vi "Extras_1SDI.vi"(8 "Scope+Safety":T3={"Safety First"={"lim reset"=FALSE, "no limit"=FALSE, "pos slew rate * dt"=100, "neg slew rate * dt"=-100, "Count(Ticks)"=0}, "Scope IPs"={"Trigger Direction"=enum."minus-plus", "Trigger Delay (ms)"=0.0, "Aquisition Rate (kHz)"=4000.0, "Trigger Offset (V)"=0.0, "Scale Offset"={"Scaling"={"Error signal"=1, "Output"=1, "DC Monitor"=1, "Threshold"=1}, "Offset"={"Error Signal"=0, "Output"=0, "DC Monitor"=0, "Threshold"=0}}}}, 11 "Extras 1SDI":T4={"Error Bit Shift "={"EPR BS"=0, "HD A x"=0, "HD A p"=0, "HD B x"=0, "HD B p"=0, "HD C x"=0, "HD C p"=0}, "I Max value"=20000, "Scan Offset"={"EPR BS"=0.0, "HD A"=0.0, "HD B"=0.0, "HD C"=0.0}, "Scan Ampl.\n     (mV)"={"EPR BS"=0.0, "HD A"=0.0, "HD B"=0.0, "HD C"=0.0}, "Scan-PII thresh"={"EPR BS"=0, "Homodyne A"=0, "Homodyne B"=0, "Homodyne C"=0}, "Re-Scan thresh"={"EPR BS"=1000, "Homodyne A"=1000, "Homodyne B"=1000, "Homodyne C"=0}, "Post-Offset"={"HD A x"=0.0, "HD A p"=0.0, "HD B x"=0.0, "HD B p"=0.0, "HD C x"=0.0, "HD C p"=0.0}}) -> (0 "Extras Homodyne C":T1, 1 "Extras Homodyne B":T1, 2 "Extras Homodyne A":T1, 3 "Extras EPR BS":T2)   [LabVIEW 2013]
uses:
  Strict Type Defs/Extras 1SDI.ctl
  Strict Type Defs/Double ISDI control.ctl
  Strict Type Defs/I16 1SDI Control.ctl
  Strict Type Defs/Scope and Safety.ctl
  Strict Type Defs/Extras PII 1SDI.ctl
  Strict Type Defs/Extras PII 1SDI HD.ctl
panel:
  in  "Extras HD C":T1
  in  "Extras HD B":T1
  in  "Extras HD A":T1
  in  "Extras PII 1SDI":T2
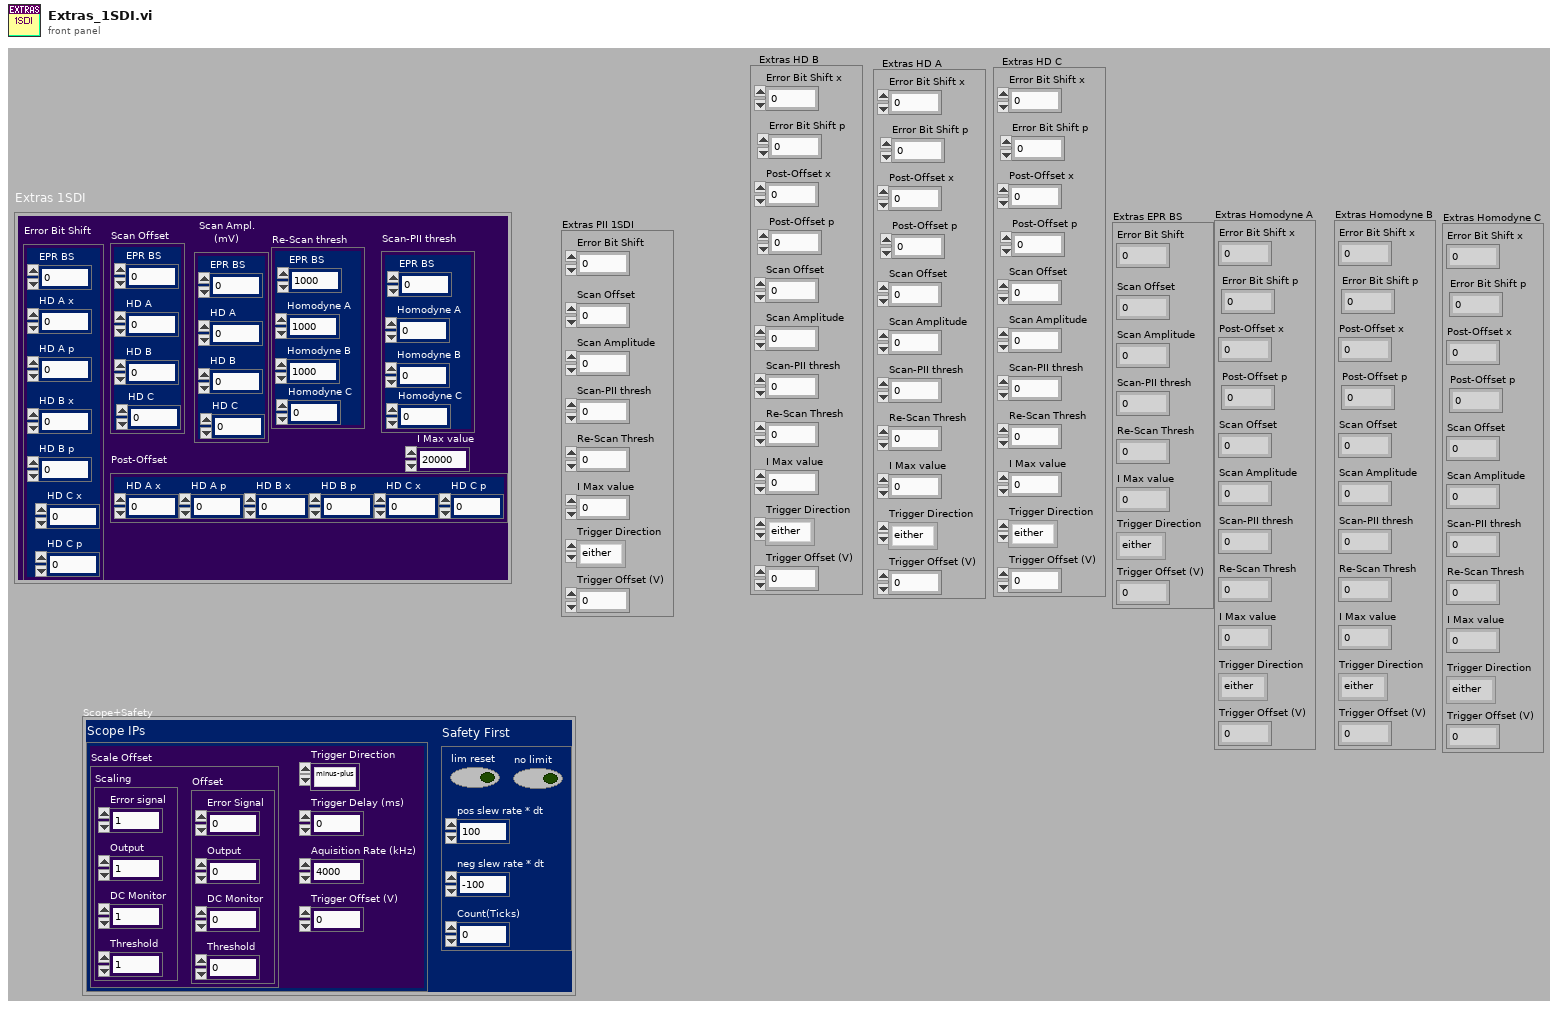
[diagram p1: front panel]
types:
  T1 = typedef "Extras PII 1SDI HD.ctl" = cluster{"Error Bit Shift p":i16, "Scan Offset":dbl, "Scan Amplitude":dbl, "Scan-PII thresh":i16, "Re-Scan Thresh":i16, "I Max value":i32, "Trigger Direction":enum8{"either", "minus-plus", "plus-minus"}, "Trigger Offset (V)":dbl, "Error Bit Shift x":i16, "Post-Offset p":dbl, "Post-Offset x":dbl}
  T2 = typedef "Extras PII 1SDI.ctl" = cluster{"Error Bit Shift":i16, "Scan Offset":dbl, "Scan Amplitude":dbl, "Scan-PII thresh":i16, "Re-Scan Thresh":i16, "I Max value":i32, "Trigger Direction":enum8{"either", "minus-plus", "plus-minus"}, "Trigger Offset (V)":dbl}
  T3 = typedef "Scope and Safety.ctl" = cluster{"Safety First":cluster{"lim reset":bool, "no limit":bool, "pos slew rate * dt":i16, "neg slew rate * dt":i16, "Count(Ticks)":u32}, "Scope IPs":cluster{"Trigger Direction":enum8{"either", "minus-plus", "plus-minus"}, "Trigger Delay (ms)":dbl, "Aquisition Rate (kHz)":dbl, "Trigger Offset (V)":dbl, "Scale Offset":cluster{"Scaling":cluster{"Error signal":i16, "Output":i16, "DC Monitor":i16, "Threshold":i16}, "Offset":cluster{"Error Signal":i16, "Output":i16, "DC Monitor":i16, "Threshold":i16}}}}
  T4 = typedef "Extras 1SDI.ctl" = cluster{"Error Bit Shift ":cluster{"EPR BS":i16, "HD A x":i16, "HD A p":i16, "HD B x":i16, "HD B p":i16, "HD C x":i16, "HD C p":i16}, "I Max value":i32, "Scan Offset":T5, "Scan Ampl.\n     (mV)":T5, "Scan-PII thresh":T6, "Re-Scan thresh":T6, "Post-Offset":cluster{"HD A x":dbl, "HD A p":dbl, "HD B x":dbl, "HD B p":dbl, "HD C x":dbl, "HD C p":dbl}}
  T5 = typedef "Double ISDI control.ctl" = cluster{"EPR BS":dbl, "HD A":dbl, "HD B":dbl, "HD C":dbl}
  T6 = typedef "I16 1SDI Control.ctl" = cluster{"EPR BS":i16, "Homodyne A":i16, "Homodyne B":i16, "Homodyne C":i16}
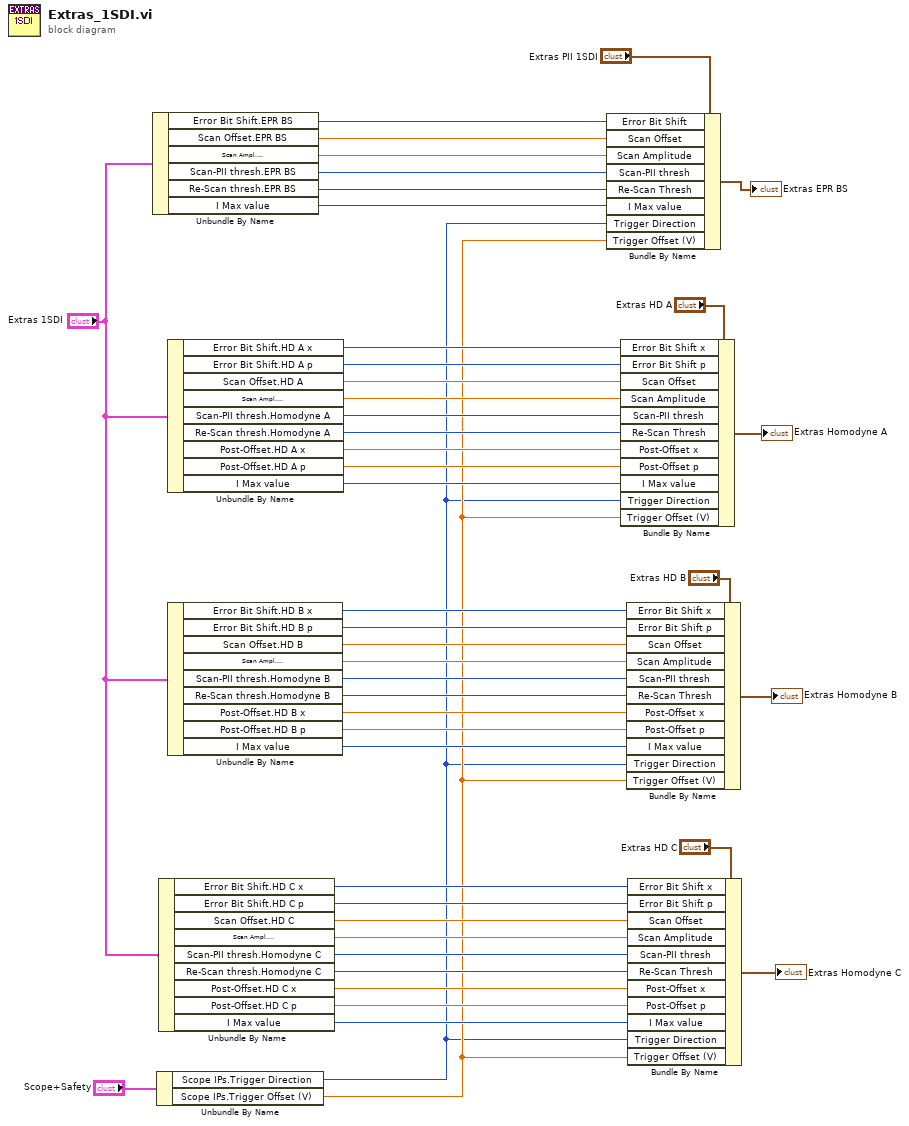
[diagram p0: block diagram]
diagram:
  n1 = Unbundle By Name("Extras 1SDI") -> ("Error Bit Shift.EPR BS"=w38:i16, "Scan Offset.EPR BS"=w37:dbl, "Scan Ampl.\n     (mV).EPR BS"=w36:dbl, "Scan-PII thresh.EPR BS"=w35:i16, "Re-Scan thresh.EPR BS"=w34:i16, "I Max value"=w33:i32)
  n2 = Unbundle By Name("Scope+Safety") -> ("Scope IPs.Trigger Direction"=w2:enum8{"either", "minus-plus", "plus-minus"}, "Scope IPs.Trigger Offset (V)"=w3:dbl)
  n3 = Unbundle By Name("Extras 1SDI") -> ("Error Bit Shift.HD C x"=w14:i16, "Error Bit Shift.HD C p"=w13:i16, "Scan Offset.HD C"=w10:dbl, "Scan Ampl.\n     (mV).HD C"=w9:dbl, "Scan-PII thresh.Homodyne C"=w8:i16, "Re-Scan thresh.Homodyne C"=w7:i16, "Post-Offset.HD C x"=w6:dbl, "Post-Offset.HD C p"=w5:dbl, "I Max value"=w4:i32)
  n4 = Unbundle By Name("Extras 1SDI") -> ("Error Bit Shift.HD A x"=w32:i16, "Error Bit Shift.HD A p"=w31:i16, "Scan Offset.HD A"=w30:dbl, "Scan Ampl.\n     (mV).HD A"=w29:dbl, "Scan-PII thresh.Homodyne A"=w28:i16, "Re-Scan thresh.Homodyne A"=w27:i16, "Post-Offset.HD A x"=w26:dbl, "Post-Offset.HD A p"=w25:dbl, "I Max value"=w24:i32)
  n5 = Unbundle By Name("Extras 1SDI") -> ("Error Bit Shift.HD B x"=w23:i16, "Error Bit Shift.HD B p"=w22:i16, "Scan Offset.HD B"=w21:dbl, "Scan Ampl.\n     (mV).HD B"=w20:dbl, "Scan-PII thresh.Homodyne B"=w19:i16, "Re-Scan thresh.Homodyne B"=w18:i16, "Post-Offset.HD B x"=w17:dbl, "Post-Offset.HD B p"=w16:dbl, "I Max value"=w15:i32)
  n6 = Bundle By Name(cluster="Extras PII 1SDI", "Error Bit Shift"=w38, "Scan Offset"=w37, "Scan Amplitude"=w36, "Scan-PII thresh"=w35, "Re-Scan Thresh"=w34, "I Max value"=w33, "Trigger Direction"=w2, "Trigger Offset (V)"=w3) -> (→"Extras EPR BS":T2)
  n7 = Bundle By Name(cluster="Extras HD A", "Error Bit Shift x"=w32, "Error Bit Shift p"=w31, "Scan Offset"=w30, "Scan Amplitude"=w29, "Scan-PII thresh"=w28, "Re-Scan Thresh"=w27, "Post-Offset x"=w26, "Post-Offset p"=w25, "I Max value"=w24, "Trigger Direction"=w2, "Trigger Offset (V)"=w3) -> (→"Extras Homodyne A":T1)
  n8 = Bundle By Name(cluster="Extras HD B", "Error Bit Shift x"=w23, "Error Bit Shift p"=w22, "Scan Offset"=w21, "Scan Amplitude"=w20, "Scan-PII thresh"=w19, "Re-Scan Thresh"=w18, "Post-Offset x"=w17, "Post-Offset p"=w16, "I Max value"=w15, "Trigger Direction"=w2, "Trigger Offset (V)"=w3) -> (→"Extras Homodyne B":T1)
  n9 = Bundle By Name(cluster="Extras HD C", "Error Bit Shift x"=w14, "Error Bit Shift p"=w13, "Scan Offset"=w10, "Scan Amplitude"=w9, "Scan-PII thresh"=w8, "Re-Scan Thresh"=w7, "Post-Offset x"=w6, "Post-Offset p"=w5, "I Max value"=w4, "Trigger Direction"=w2, "Trigger Offset (V)"=w3) -> (→"Extras Homodyne C":T1)
